vi "ReaddNoise.vi"(1 "Data in":i16[][](array[numeric])=[[1, 2, 2, 3, 4], [2, 3, 3, 0, 0], [1, 1, 2, 3, 4]]) -> (0 "Data out":i16[][](array[numeric]))   [LabVIEW 2022 SP3]
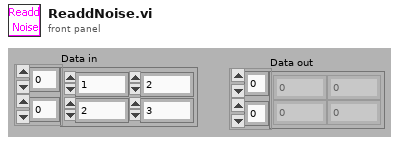
[diagram p1: front panel]
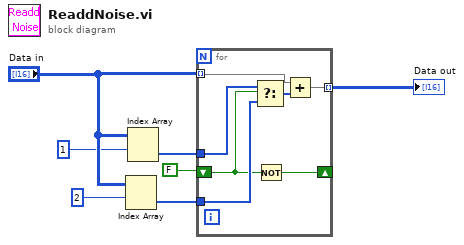
[diagram p0: block diagram]
diagram:
  n1 = Index Array(array="Data in", index (row)=2) -> (element=w5:i16[])  [unwired: 1 in]
  n2 = Index Array(array="Data in", index (row)=1) -> (element=w6:i16[])  [unwired: 1 in]
  n3 = for {
    tunnel: "Data in" -> [w11] mode=indexing
    tunnel: w6 -> [w14]
    tunnel: w5 -> [w13]
    tunnel: [w10] -> w4 mode=indexing
    shift-right: [w8] -> _
    shift-left: FALSE -> [w9]
    n4 = Select(t=w14, s=w9, f=w13) -> (s? t:f=w12:i16[])
    n5 = Not(x=w9) -> (.not. x?=w8:bool)
    n6 = Add(x=w11, y=w12) -> (x+y=w10:i16[])
  }
  "Data out" <- w4
